vi "获取特殊符号.vi"() -> ()   [LabVIEW 2012]
panel:
  out "特殊符号（菜单）":u16(ring)=8 items=["＃", "＠", "＆", "＊", "※", "§", "〃", "№", "〓", "○", "●", "△", "▲", "◎", "☆", "★", "◇", "◆", "□", "■", "▽", "▼", "㊣", "℅", "ˉ", "￣", "＿", "﹉", "﹊", "﹍", "﹎", "﹋", "﹌", "﹟", "﹠", "﹡", "♀", "♂", "⊕", "⊙", "↑", "↓", "←", "→", "↖", "↗", "↙", "↘", "∥", "∣", "／", "＼", "∕﹨"]
  out "特殊符号":u16(ring)=10 items=["＃", "＠", "＆", "＊", "※", "§", "〃", "№", "〓", "○", "●", "△", "▲", "◎", "☆", "★", "◇", "◆", "□", "■", "▽", "▼", "㊣", "℅", "ˉ", "￣", "＿", "﹉", "﹊", "﹍", "﹎", "﹋", "﹌", "﹟", "﹠", "﹡", "♀", "♂", "⊕", "⊙", "↑", "↓", "←", "→", "↖", "↗", "↙", "↘", "∥", "∣", "／", "＼", "∕﹨"]
  out "特殊符号":string[](array[string])=["＃", "＠", "＆", "＊", "※", "§", "〃", "№", "〓", "○", "●", "△", "▲", "◎", "☆", "★", "◇", "◆", "□", "■", "▽", "▼", "㊣", "℅", "ˉ", "￣", "＿", "﹉", "﹊", "﹍", "﹎", "﹋", "﹌", "﹟", "﹠", "﹡", "♀", "♂", "⊕", "⊙", "↑", "↓", "←", "→", "↖", "↗", "↙", "↘", "∥", "∣", "／", "＼", "∕﹨"]
  in  "特殊符号":string="＃ ＠ ＆ ＊ ※ § 〃 № 〓 ○ ● △ ▲ ◎ ☆ ★ ◇ ◆ □ ■ ▽ ▼ ㊣ ℅ ˉ ￣ ＿ ﹉ ﹊ ﹍ ﹎ ﹋ ﹌ ﹟ ﹠ ﹡ ♀ ♂ ⊕ ⊙ ↑ ↓ ← → ↖ ↗ ↙ ↘ ∥ ∣ ／ ＼ ∕﹨"
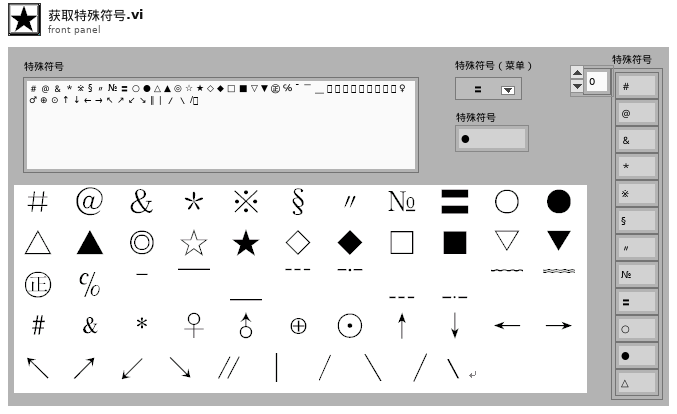
[diagram p1: front panel]
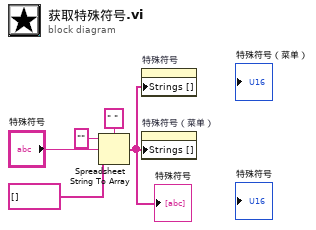
[diagram p0: block diagram]
diagram:
  n1 = Spreadsheet String To Array(delimiter (Tab)=" " ("分隔符(Tab)"), format string="" ("格式字符串"), spreadsheet string="特殊符号", array type (2D Dbl)=string[] []) -> (array=w1:string[])
  "特殊符号" <- w1
  n2 = property on="特殊符号" class="Ring (严格)"("Strings []"=w1) -> ()  [unwired: 2 in, 2 out]
  n3 = property on="特殊符号（菜单）" class="Ring (严格)"("Strings []"=w1) -> ()  [unwired: 2 in, 2 out]
